vi "战舰移动.vi"() -> ()   [LabVIEW 2018]
panel:
  out "战舰":T1
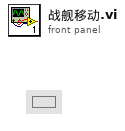
[diagram p1: front panel]
types:
  T1 = typedef "战列巡洋舰.ctl" = picture
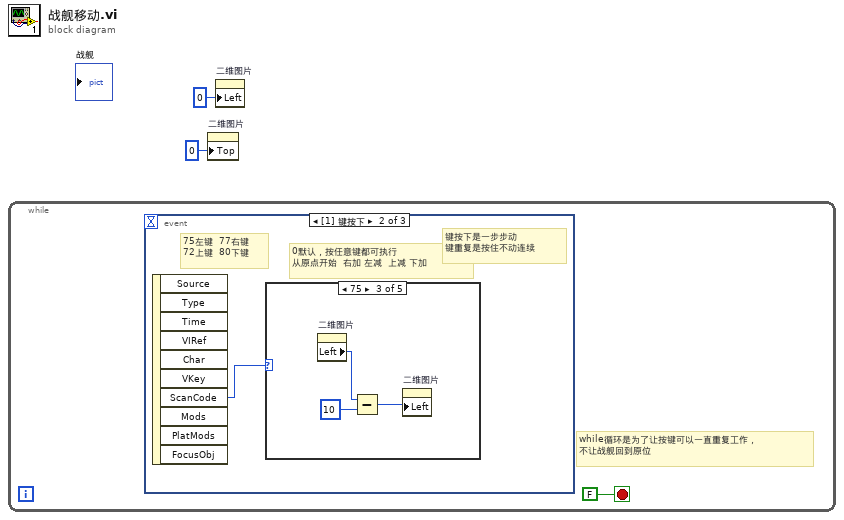
[diagram p0: block diagram]
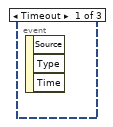
[diagram p2: hidden frame]
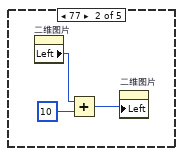
[diagram p4: hidden frame]
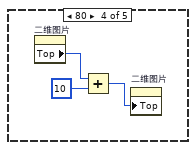
[diagram p5: hidden frame]
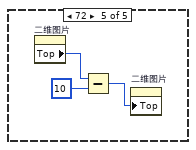
[diagram p6: hidden frame]
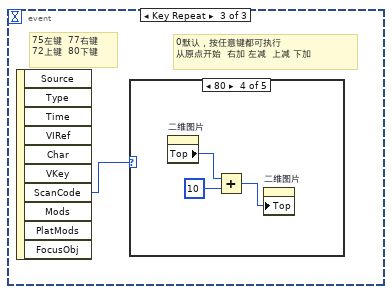
[diagram p7: hidden frame]
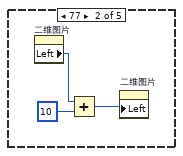
[diagram p9: hidden frame]
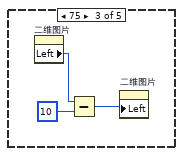
[diagram p10: hidden frame]
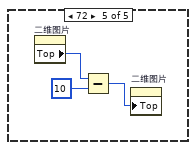
[diagram p11: hidden frame]
diagram:
  n1 = while {
    stop <- FALSE stop-if-true
    # "while循环是为了让按键可以一直重复工作，\n不让战舰回到原位"
    n2 = event shown="[1] 键按下" {
      selector: _ -> [_ _ _]
      dyn-events: _ -> [_ _ _]
      timeout: _ -> [_ _ _]
      event Timeout {
        n3 = event-data() -> ()  [unwired: 1 in, 3 out]
      }
      event Key Down {
        # "键按下是一步步动\n键重复是按住不动连续"
        # "75左键  77右键\n72上键  80下键"
        # "0默认，按任意键都可执行\n从原点开始  右加 左减  上减 下加"
        n4 = event-data() -> ("ScanCode"=w4:i16)  [unwired: 1 in, 9 out]
        n5 = case shown="75" w4 {
          frame 0, Default {
          }
          frame 77 {
            n6 = property on="二维图片" class="Pict (严格)"() -> ("Left"=w7:i32)  [unwired: 2 in, 2 out]
            n7 = Add(x=w7, y=10) -> (x+y=w6:i32)
            n8 = property on="二维图片" class="Pict (严格)"("Left"=w6) -> ()  [unwired: 2 in, 2 out]
          }
          frame 75 {
            n9 = property on="二维图片" class="Pict (严格)"() -> ("Left"=w10:i32)  [unwired: 2 in, 2 out]
            n10 = Subtract(x=w10, y=10) -> (x-y=w9:i32)
            n11 = property on="二维图片" class="Pict (严格)"("Left"=w9) -> ()  [unwired: 2 in, 2 out]
          }
          frame 80 {
            n12 = property on="二维图片" class="Pict (严格)"() -> ("Top"=w12:i32)  [unwired: 2 in, 2 out]
            n13 = Add(x=w12, y=10) -> (x+y=w11:i32)
            n14 = property on="二维图片" class="Pict (严格)"("Top"=w11) -> ()  [unwired: 2 in, 2 out]
          }
          frame 72 {
            n15 = property on="二维图片" class="Pict (严格)"() -> ("Top"=w16:i32)  [unwired: 2 in, 2 out]
            n16 = Subtract(x=w16, y=10) -> (x-y=w15:i32)
            n17 = property on="二维图片" class="Pict (严格)"("Top"=w15) -> ()  [unwired: 2 in, 2 out]
          }
        }
      }
      event Key Repeat {
        # "75左键  77右键\n72上键  80下键"
        # "0默认，按任意键都可执行\n从原点开始  右加 左减  上减 下加"
        n18 = event-data() -> ("ScanCode"=w17:i16)  [unwired: 1 in, 9 out]
        n19 = case shown="80" w17 {
          frame 0, Default {
          }
          frame 77 {
            n20 = property on="二维图片" class="Pict (严格)"() -> ("Left"=w20:i32)  [unwired: 2 in, 2 out]
            n21 = Add(x=w20, y=10) -> (x+y=w19:i32)
            n22 = property on="二维图片" class="Pict (严格)"("Left"=w19) -> ()  [unwired: 2 in, 2 out]
          }
          frame 75 {
            n23 = property on="二维图片" class="Pict (严格)"() -> ("Left"=w23:i32)  [unwired: 2 in, 2 out]
            n24 = Subtract(x=w23, y=10) -> (x-y=w22:i32)
            n25 = property on="二维图片" class="Pict (严格)"("Left"=w22) -> ()  [unwired: 2 in, 2 out]
          }
          frame 80 {
            n26 = property on="二维图片" class="Pict (严格)"() -> ("Top"=w25:i32)  [unwired: 2 in, 2 out]
            n27 = Add(x=w25, y=10) -> (x+y=w24:i32)
            n28 = property on="二维图片" class="Pict (严格)"("Top"=w24) -> ()  [unwired: 2 in, 2 out]
          }
          frame 72 {
            n29 = property on="二维图片" class="Pict (严格)"() -> ("Top"=w29:i32)  [unwired: 2 in, 2 out]
            n30 = Subtract(x=w29, y=10) -> (x-y=w28:i32)
            n31 = property on="二维图片" class="Pict (严格)"("Top"=w28) -> ()  [unwired: 2 in, 2 out]
          }
        }
      }
    }
  }
  n32 = property on="二维图片" class="Pict (严格)"("Top"=0 ("位置:置顶")) -> ()  [unwired: 2 in, 2 out]
  n33 = property on="二维图片" class="Pict (严格)"("Left"=0 ("位置:居左")) -> ()  [unwired: 2 in, 2 out]
